vi "getFTData.vi"(5 "error in":errorcluster, 6 "bias":dbl, 7 "Timing parameters":T1={"Sample Rate"=1000.0, "Samples to Read"=100}, 8 "task in":refnum<k21>) -> (0 "error out":errorcluster, 1 "Force":dbl[](array[numeric]), 2 "Voltage":dbl[](array[numeric]), 3 "task out 2":refnum<k21>)   [LabVIEW 2012]
uses:
  <vilib>/DAQmx/read.llb/DAQmx Read (Analog 1D DBL 1Chan NSamp).vi
  <vilib>/DAQmx/miscellaneous.llb/DAQmx Fill In Error Info.vi
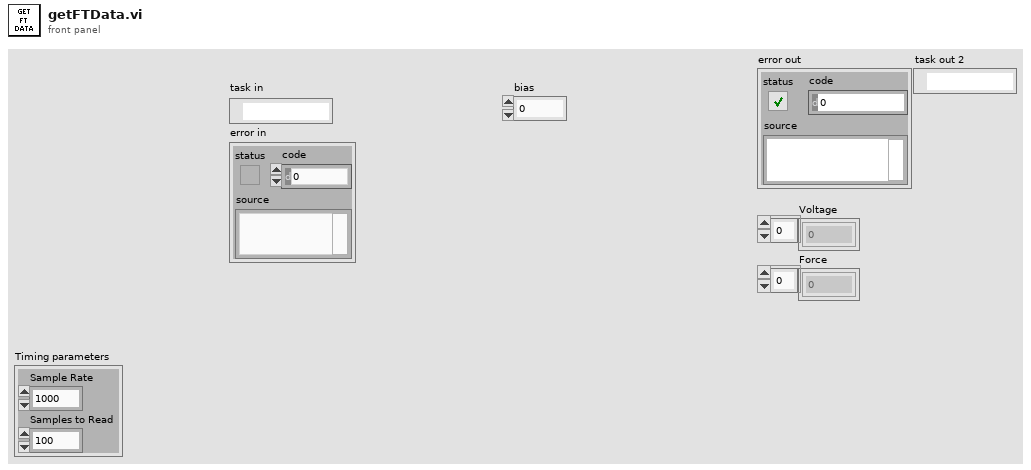
[diagram p1: front panel]
types:
  T1 = cluster{"Sample Rate":dbl, "Samples to Read":i32}
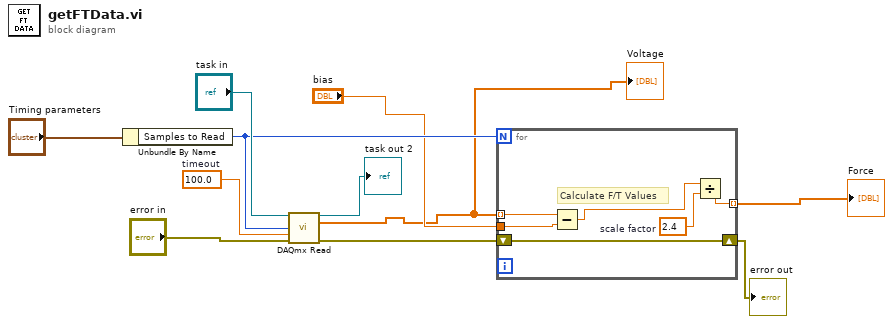
[diagram p0: block diagram]
diagram:
  w5 = 100.0  # timeout
  n1 = Unbundle By Name("Timing parameters") -> ("Samples to Read"=w8:i32)
  n2 = call-poly <vilib>:"DAQmx Read.vi"("task/channels in"="task in", "number of samples per channel"=w8, "timeout"=w5, "error in"="error in") -> ("task out"=→"task out 2":refnum<k21>, "data"=w1:dbl[], "error out"=w4:errorcluster)  [unwired: 9 in]
  "Voltage" <- w1
  n3 = for {
    N: w8 -> [_]
    tunnel: [w13] -> w2 mode=indexing
    shift-right: [w16] -> w6
    shift-left: w4 -> [w16]
    tunnel: w1 -> [w17] mode=indexing
    tunnel: "bias" -> [w15]
    w14 = 2.4  # scale factor
    # "Calculate F/T Values"
    n4 = Subtract(x=w17, y=w15) -> (x-y=w12:dbl)
    n5 = Divide(x=w12, y=w14) -> (x/y=w13:dbl)
  }
  "error out" <- w6
  "Force" <- w2
